vi "Do Core.vi"(8 "error in (no error)":errorcluster, 9 "Actor in":refnum<class "Actor.lvclass">, 11 "Reply Message":refnum<class "Get Proxy Enq Msg.lvclass">) -> (0 "error out":errorcluster, 1 "Actor out":refnum<class "Actor.lvclass">, 2 "Reply":variant)   [LabVIEW 2014, in "Target.lvlib" / "Get Proxy Enq Msg.lvclass"]
doc: "(<B>Filename</B>: Actor Framework.lvlib:Reply Msg.lvclass:Do Core.vi)\n\nDefines what an actor does when it receives <B>Reply Message</B>. This method also defines the <B>Reply</B> that is returned to the actor that sent <B>Reply Message</B>.\n\nBy default, this method does nothing, and <B>Reply</B> is the ancestor Message class. A child class must override this method to define behavior and specify a child of the Message class to return in the <B>Reply</B> output."
uses:
  Get Proxy Enq Msg.lvclass
  <vilib>/ActorFramework/Actor/Actor.lvclass
  Target/Target.lvclass
  Target/Target.lvclass/Target.ctl
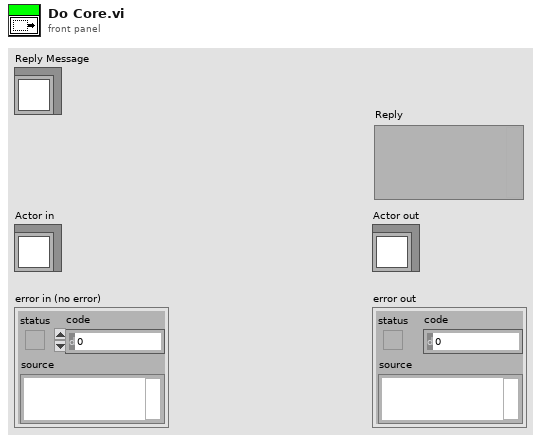
[diagram p1: front panel]
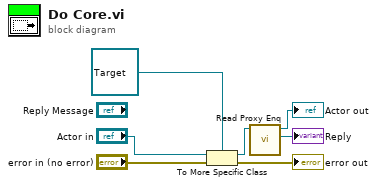
[diagram p0: block diagram]
diagram:
  n1 = To More Specific Class(target class=refnum<class "Target.lvclass"> refnum ("Target.lvlib:Target.lvclass"), reference="Actor in", error in="error in (no error)") -> (specific class reference=w4:refnum<class "Target.lvclass">, error out=→"error out":errorcluster)
  n2 = call "Read Proxy Enq.vi"("Target in"=w4) -> ("Actor Framework:Message Enqueuer"=→"Reply":refnum<class "Message Enqueuer.lvclass">, "Target out"=→"Actor out":refnum<class "Target.lvclass">)  [unwired: 9 in]
